vi "Parse Global Vars-Channel Names.vi"(10 "2D Sensor Info":string[][](array[string]), 11 "Data":T2) -> (1 "Data Array":dbl[][](array[numeric]), 2 "Channel Names Array":string[](array[string]), 3 "Timestamp Array":timestamp[](array[timestamp]))   [LabVIEW 2018]
doc: "Takes in the global variables and parses it according to the used channels in the APU file. Outputs two same-sized arrays for channels names and data."
uses:
  File IO.lvlib
  Top Level/Shared Controls/Acq Data.ctl
  Top Level/Shared Controls/All Data Cluster.ctl
  Top Level/Shared Controls/Analyzed Data Sets.ctl
  Top Level/Shared Controls/Parsed Tag Cluster.ctl
panel:
  out "Good Tags":T1[](array[typedef])
  out "[Parsed Tags]":T1[](array[typedef])
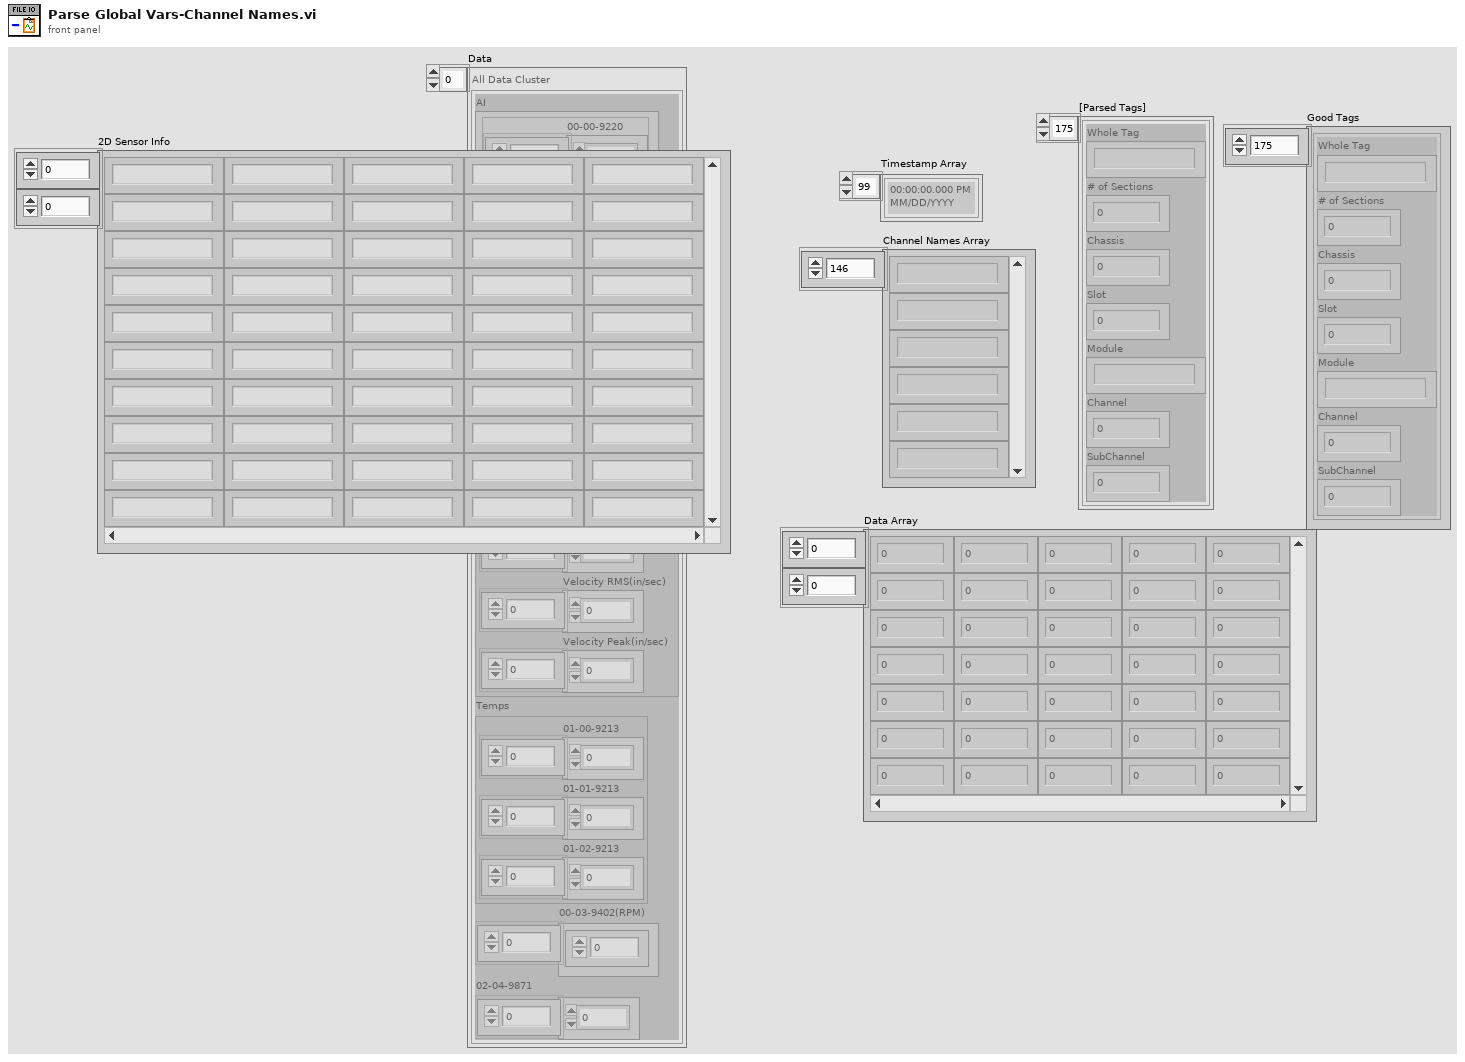
[diagram p1: front panel]
types:
  T1 = typedef "Parsed Tag Cluster.ctl" = cluster{"Whole Tag":string, "# of Sections":u8, "Chassis":u8, "Slot":u8, "Module":string, "Channel":u8, "SubChannel":u8}
  T2 = typedef "Analyzed Data Sets.ctl" = T3[]
  T3 = typedef "All Data Cluster.ctl" = cluster{"AI":T4, "Accel Data":cluster{"Accel RMS(in/sec2)":dbl[], "Accel Peak(in/sec2)":dbl[], "Velocity RMS(in/sec)":dbl[], "Velocity Peak(in/sec)":dbl[]}, "Temps":cluster{"01-00-9213":dbl[], "01-01-9213":dbl[], "01-02-9213":dbl[]}, "00-03-9402(RPM)":dbl[], "02-04-9871":dbl[]}
  T4 = typedef "Acq Data.ctl" = cluster{"00-00-9220":dbl[], "00-01-9220":dbl[], "02-02-9219":dbl[], "02-03-9227":dbl[], "02-05-9205":dbl[]}
  T5 = cluster{"00-00-9205 Calib":dbl[], "00-01-9205 Calib":dbl[], "01-00-9213 Calib":dbl[], "01-01-9213 Calib":dbl[], "01-02-9213 Calib":dbl[], "02-02-9219 Calib":dbl[], "02-03-9227 Calib":dbl[], "00-02-9234 Calib":dbl[], "00-03-9402 Calib":dbl[], "02-05-9205 Calib":dbl[], "02-04-9871-00":dbl[]}
  T6 = typedef "Calculated Data.ctl" = cluster{"C.00":dbl, "C.01":dbl, "C.02":dbl, "C.03":dbl, "C.04":dbl, "C.05":dbl, "C.06":dbl, "C.07":dbl, "C.08":dbl, "C.09":dbl, "C.10":dbl, "C.11":dbl, "C.12":dbl, "C.13":dbl, "C.14":dbl, "C.15":dbl, "C.16":dbl, "C.17":dbl, "C.18":dbl, "C.19":dbl, "C.20":dbl, "C.21":dbl, "C.22":dbl, "C.23":dbl, "C.24":dbl, "C.25":dbl, "C.26":dbl, "C.27":dbl, "C.28":dbl, "C.29":dbl, "C.30":dbl, "C.31":dbl, "C.32":dbl, "C.33":dbl, "C.34":dbl, "C.35":dbl, "C.36":dbl, "C.37":dbl, "C.38":dbl, "C.39":dbl, "C.40":dbl, "C.41":dbl, "C.42":dbl, "C.43":dbl, "C.44":dbl, "C.45":dbl, "C.46":dbl, "C.47":dbl, "C.48":dbl, "C.49":dbl, "C.50":dbl, "C.51":dbl, "C.52":dbl, "C.53":dbl, "C.54":dbl, "C.55":dbl, "C.56":dbl}
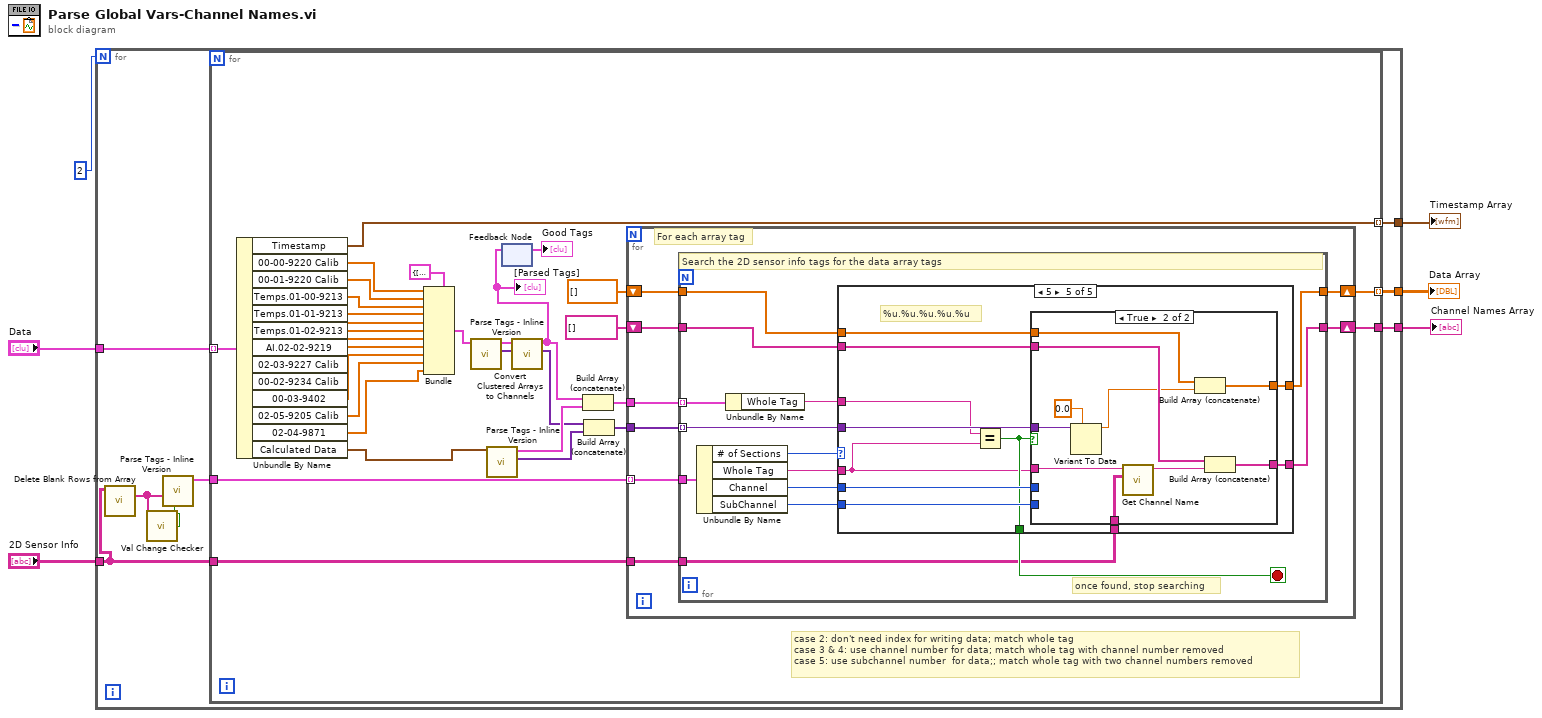
[diagram p0: block diagram]
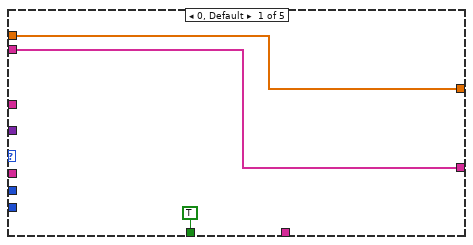
[diagram p2: hidden frame]
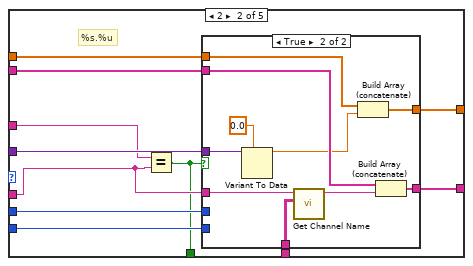
[diagram p3: hidden frame]
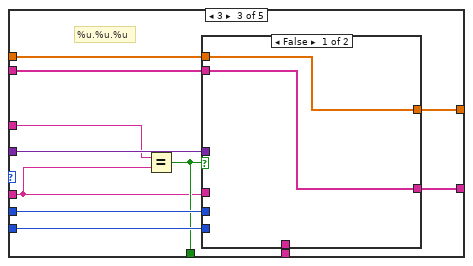
[diagram p5: hidden frame]
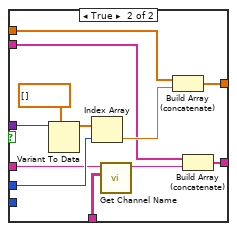
[diagram p6: hidden frame]
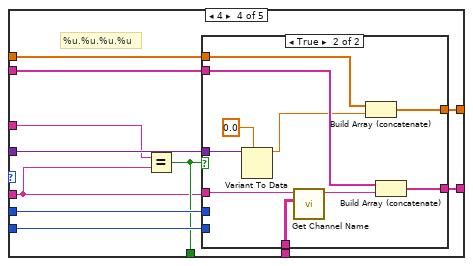
[diagram p7: hidden frame]
diagram:
  n1 = for {
    N: 2 -> [_]
    tunnel: "2D Sensor Info" -> [w13]
    tunnel: [w12] -> w5
    tunnel: [w11] -> w4
    tunnel: [w10] -> w1
    tunnel: "Data" -> [w9]
    n2 = call "Delete Blank Rows from Array.vi"("2D Array In"=w13) -> ("All Used Channel Tags"=w8:string[])  [unwired: 8 in, 2 out]
    n3 = call "Val Change Checker.vi"("Current Value in"=w8) -> ("Value Change?"=w7:bool)
    n4 = call "Parse Tags - Inline Version.vi"("New Tag Info (F)"=w7, "[Tags]"=w8) -> ("[Parsed Tags]"=w14:T1[])  [unwired: 6 in, 3 out]
    n5 = for {
      tunnel: w9 -> [w39] mode=indexing
      tunnel: w13 -> [w27]
      tunnel: [w25] -> w10
      tunnel: w14 -> [w19]
      tunnel: [w24] -> w12 mode=indexing
      tunnel: [w23] -> w11 mode=indexing
      # "case 2: don't need index for writing data; match whole tag\ncase 3 & 4: use channel number for data; match whole tag with channel number removed\ncase 5: use subchannel number  for data;; match whole tag with two channel numbers removed"
      n6 = Unbundle By Name(w39) -> ("Timestamp"=w23:timestamp, "00-00-9220 Calib"=w38:dbl[], "00-01-9220 Calib"=w37:dbl[], "Temps.01-00-9213"=w36:dbl[], "Temps.01-01-9213"=w35:dbl[], "Temps.01-02-9213"=w34:dbl[], "AI.02-02-9219"=w33:dbl[], "02-03-9227 Calib"=w32:dbl[], "00-02-9234 Calib"=w31:dbl[], "00-03-9402"=w30:dbl[], "02-05-9205 Calib"=w29:dbl[], "02-04-9871"=w15:dbl[], "Calculated Data"=w28:T6)
      n7 = Bundle(cluster=T5 {"00-00-9205 Calib"=[], "00-01-9205 Calib"=[], "01-00-9213 Calib"=[], "01-01-9213 Calib"=[], "01-02-9213 Calib"=[], "02-02-9219 Calib"=[], "02-03-9227 Calib"=[], "00-02-9234 Calib"=[], "00-03-9402 Calib"=[], "02-05-9205 Calib"=[], "02-04-9871-00"=[]} ("output cluster"), "00-00-9205 Calib"=w38, "00-01-9205 Calib"=w37, "01-00-9213 Calib"=w36, "01-01-9213 Calib"=w35, "01-02-9213 Calib"=w34, "02-02-9219 Calib"=w33, "02-03-9227 Calib"=w32, "00-02-9234 Calib"=w31, "00-03-9402 Calib"=w30, "02-05-9205 Calib"=w29, "02-04-9871-00"=w15) -> (w45:T5)
      n8 = call "Parse Tags - Inline Version.vi"("Cluster of Controls"=w45) -> ("[VData out]"=w22:variant[], "[Parsed Tags]"=w18:T1[])  [unwired: 7 in, 2 out]
      n9 = call "Parse Tags - Inline Version.vi"("Cluster of Controls"=w28) -> ("[VData out]"=w42:variant[], "[Parsed Tags]"=w44:T1[])  [unwired: 7 in, 2 out]
      n10 = feedback #1() -> (→"Good Tags":T1[])  [unwired: 1 in]
      n11 = call "Convert Clustered Arrays to Channels.vi"("[VData out]"=w22, "[Parsed Tags]"=w18) -> ("[VData out]"=w21:variant[], "[Parsed Tags]"=w16:T1[])  [unwired: 6 in, 2 out]
      "[Parsed Tags]" <- w16
      n12 = feedback-in #1(w16) -> ()
      n13 = Build Array (concatenate)(w16, w44) -> (w43:T1[])
      n14 = Build Array (concatenate)(w21, w42) -> (w41:variant[])
      n15 = for {
        tunnel: w41 -> [w53]
        tunnel: w19 -> [w52] mode=indexing
        tunnel: w43 -> [w51]
        shift-right: [w49] -> w24
        shift-left: dbl[] [] ("Data Array") -> [w50]
        tunnel: w27 -> [w48]
        shift-right: [w47] -> w25
        shift-left: string[] [] ("array") -> [w46]
        # "For each array tag"
        n16 = for {
          tunnel: w53 -> [w67] mode=indexing
          tunnel: w52 -> [w65]
          tunnel: w51 -> [w66] mode=indexing
          tunnel: w48 -> [w56]
          tunnel: w46 -> [w54]
          tunnel: [w55] -> w47
          tunnel: w50 -> [w58]
          tunnel: [w57] -> w49
          stop <- w64 stop-if-true
          # "once found, stop searching"
          # "Search the 2D sensor info tags for the data array tags"
          n17 = Unbundle By Name(w65) -> ("# of Sections"=w60:u8, "Whole Tag"=w63:string, "Channel"=w62:u8, "SubChannel"=w61:u8)
          n18 = Unbundle By Name(w66) -> ("Whole Tag"=w59:string)
          n19 = case shown="5" w60 {
            tunnel: w67 -> [_ w81 w104 w129 w152]
            tunnel: [w69 w80 w103 w128 w151] -> w57
            tunnel: [TRUE w71 w95 w120 w143] -> w64
            tunnel: w59 -> [_ w73 w96 w121 w144]
            tunnel: w63 -> [_ w72 w94 w119 w142]
            tunnel: w62 -> [_ w79 w102 w127 w150]
            tunnel: w61 -> [_ w78 w101 w126 w149]
            tunnel: w58 -> [w69 w77 w100 w125 w148]
            tunnel: w56 -> [_ w76 w99 w124 w147]
            tunnel: [w68 w75 w98 w123 w146] -> w55
            tunnel: w54 -> [w68 w74 w97 w122 w145]
            frame 0, Default {
            }
            frame 2 {
              # "%s.%u"
              n20 = Equal?(x=w73, y=w72) -> (x = y?=w71:bool)
              n21 = case shown="True" w71 {
                tunnel: w81 -> [_ w93]
                tunnel: [w83 w91] -> w80
                tunnel: w79 -> [_ _]
                tunnel: w78 -> [_ _]
                tunnel: w77 -> [w83 w92]
                tunnel: w72 -> [_ w89]
                tunnel: w76 -> [_ w90]
                tunnel: [w82 w87] -> w75
                tunnel: w74 -> [w82 w86]
                frame False {
                }
                frame True {
                  n22 = Variant To Data(type=0.0, Variant=w93) -> (data=w84:dbl)  [unwired: 1 in, 1 out]
                  n23 = call "Get Channel Name.vi"("2D Sensor Info"=w90, "Whole Tag"=w89) -> ("Channel Name (Units)"=w88:string)  [unwired: 9 in]
                  n24 = Build Array (concatenate)(w92, w84) -> (w91:dbl[])
                  n25 = Build Array (concatenate)(w86, w88) -> (w87:string[])
                }
              }
            }
            frame 3 {
              # "%u.%u.%u"
              n26 = Equal?(x=w96, y=w94) -> (x = y?=w95:bool)
              n27 = case shown="False" w95 {
                tunnel: w104 -> [_ w118]
                tunnel: [w106 w113] -> w103
                tunnel: w102 -> [_ w112]
                tunnel: w101 -> [_ _]
                tunnel: w100 -> [w106 w115]
                tunnel: w94 -> [_ w110]
                tunnel: w99 -> [_ w111]
                tunnel: [w105 w108] -> w98
                tunnel: w97 -> [w105 w107]
                frame False {
                }
                frame True {
                  n28 = Variant To Data(type=dbl[] [], Variant=w118) -> (data=w116:dbl[])  [unwired: 1 in, 1 out]
                  n29 = Index Array(array=w116, index=w112) -> (element=w114:dbl)
                  n30 = call "Get Channel Name.vi"("2D Sensor Info"=w111, "Whole Tag"=w110) -> ("Channel Name (Units)"=w109:string)  [unwired: 9 in]
                  n31 = Build Array (concatenate)(w115, w114) -> (w113:dbl[])
                  n32 = Build Array (concatenate)(w107, w109) -> (w108:string[])
                }
              }
            }
            frame 4 {
              # "%u.%u.%u.%u"
              n33 = Equal?(x=w121, y=w119) -> (x = y?=w120:bool)
              n34 = case shown="True" w120 {
                tunnel: w129 -> [_ w141]
                tunnel: [w131 w139] -> w128
                tunnel: w127 -> [_ _]
                tunnel: w126 -> [_ _]
                tunnel: w125 -> [w131 w140]
                tunnel: w119 -> [_ w137]
                tunnel: w124 -> [_ w138]
                tunnel: [w130 w135] -> w123
                tunnel: w122 -> [w130 w134]
                frame False {
                }
                frame True {
                  n35 = Variant To Data(type=0.0, Variant=w141) -> (data=w132:dbl)  [unwired: 1 in, 1 out]
                  n36 = call "Get Channel Name.vi"("2D Sensor Info"=w138, "Whole Tag"=w137) -> ("Channel Name (Units)"=w136:string)  [unwired: 9 in]
                  n37 = Build Array (concatenate)(w140, w132) -> (w139:dbl[])
                  n38 = Build Array (concatenate)(w134, w136) -> (w135:string[])
                }
              }
            }
            frame 5 {
              # "%u.%u.%u.%u.%u"
              n39 = Equal?(x=w144, y=w142) -> (x = y?=w143:bool)
              n40 = case shown="True" w143 {
                tunnel: w152 -> [_ w164]
                tunnel: [w154 w162] -> w151
                tunnel: w150 -> [_ _]
                tunnel: w149 -> [_ _]
                tunnel: w148 -> [w154 w163]
                tunnel: w142 -> [_ w160]
                tunnel: w147 -> [_ w161]
                tunnel: [w153 w158] -> w146
                tunnel: w145 -> [w153 w157]
                frame False {
                }
                frame True {
                  n41 = Variant To Data(type=0.0, Variant=w164) -> (data=w155:dbl)  [unwired: 1 in, 1 out]
                  n42 = call "Get Channel Name.vi"("2D Sensor Info"=w161, "Whole Tag"=w160) -> ("Channel Name (Units)"=w159:string)  [unwired: 9 in]
                  n43 = Build Array (concatenate)(w163, w155) -> (w162:dbl[])
                  n44 = Build Array (concatenate)(w157, w159) -> (w158:string[])
                }
              }
            }
          }
        }
      }
    }
  }
  "Data Array" <- w5
  "Channel Names Array" <- w1
  "Timestamp Array" <- w4
